vi "EDIT USER IN PGSQL.vi"(8 "USER/ITEM DATA TRANSFER IN":T2(array[cluster]), 9 "REFERENCES":T3, 10 "USER INFO IN":T4, 11 "Image In":T1) -> (0 "USER/ITEM DATA TRANSFER OUT":T2(array[cluster]), 2 "USER INFO OUT":T4)   [LabVIEW 2019]
uses:
  Controls/References Cluster.ctl
  <vilib>/userDefined/High Color/IMAQdx.ctl
  Controls/Custom Calendar/Custom Calendar.xctl
  <vilib>/vision/Image Controls.llb/IMAQ Image.ctl
  Controls/Table Data Types/User Data Type.ctl
  <vilib>/addons/database/Connection.llb/DB Tools Open Connec (String).vi
  <vilib>/addons/database/Connection.llb/Conn Execute.vi
  <vilib>/addons/database/Recordset.llb/Rec Destroy - Connection.vi
  <vilib>/addons/database/NI_Database_API.lvlib
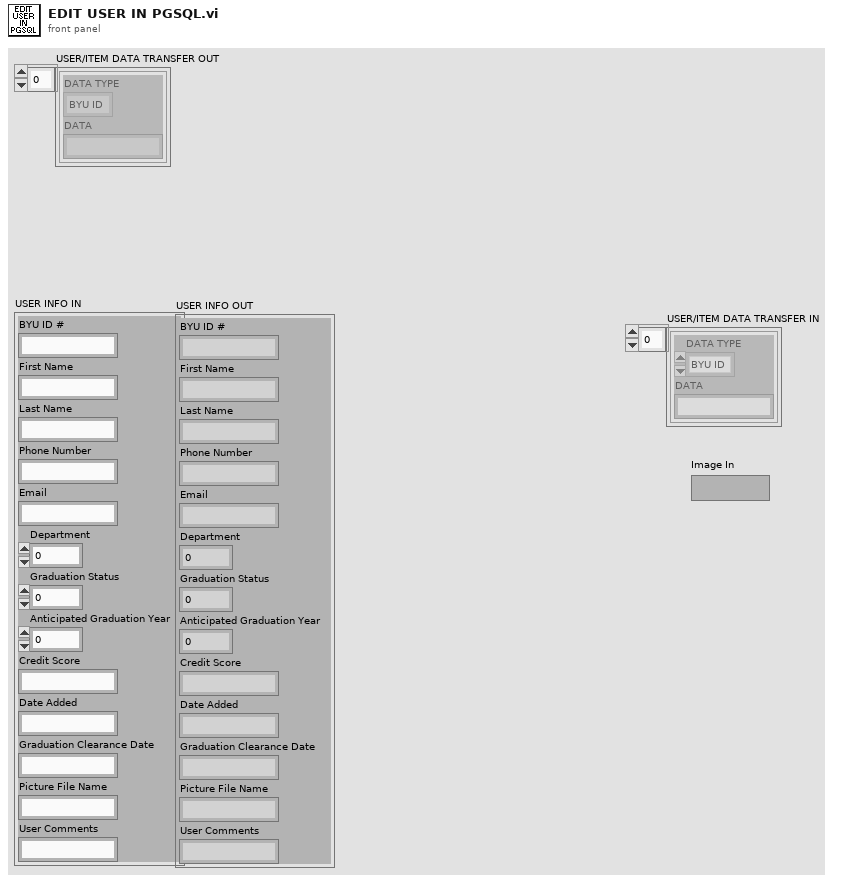
[diagram p1: front panel]
types:
  T1 = typedef "IMAQ Image.ctl" = refnum<image>
  T2 = cluster{"DATA TYPE":enum16{"BYU ID", "ME#/IDENTIFIER", "BYU ICN"}, "DATA":string}[]
  T3 = typedef "References Cluster.ctl" = cluster{"MAIN PAGES":refnum<vi>, "ADD/EDIT ITEM REFERENCES":cluster{"Identifier":refnum<vi>, "BYU ICN #":refnum<vi>, "Item Description":refnum<vi>, "Comments":refnum<vi>, "Checked Out Date":refnum<vi>, "Due Date":refnum<vi>, "Check Out Location":refnum<vi>, "Reminder Count":refnum<vi>, "Most Recent Reminder Date":refnum<vi>, "BYU ID #":refnum<vi>, "Building/Room":refnum<vi>, "Location in Room":refnum<vi>, "Manual":refnum<vi>, "Manufacturer":refnum<vi>, "Model #":refnum<vi>, "Serial #":refnum<vi>, "Date Acquired":refnum<vi>, "ADD/EDIT ITEM LABEL":refnum<vi>, "ARCHIVE ITEM":refnum<vi>, "Archive Item Inputs":refnum<vi>, "Reminder Notes":refnum<vi>}, "ADD/EDIT USER REFERENCES":cluster{"BYU ID # (##-###-####)":refnum<vi>, "First Name":refnum<vi>, "Last Name":refnum<vi>, "Phone Number (###-###-####)":refnum<vi>, "Email":refnum<vi>, "Department":refnum<vi>, "Graduation Status":refnum<vi>, "Anticipated Graduation Year":refnum<vi>, "Credit Score":refnum<vi>, "Date Added":refnum<vi>, "Graduation Clearance Date":refnum<vi>, "Picture File Name":refnum<vi>, "ADD/EDIT USER LABEL":refnum<vi>, "Department Map":refnum<vi>, "Status Map":refnum<vi>, "Anticipated Graduation Year Map":refnum<vi>, "User Agreement":refnum<vi>, "User Comments":refnum<vi>, "Camera":refnum<vi>}, "RETURN ITEM REFERENCES":cluster{"Item or Person:":refnum<vi>, "Search Return Results":refnum<vi>, "What are you searching for?":refnum<vi>}, "SEARCH DATABASE REFERENCES":cluster{"What to Search For:":refnum<vi>, "Where to Search":refnum<vi>, "Column to Search In":refnum<vi>, "Column to Sort By":refnum<vi>, "Search Database Results":refnum<vi>, "Inventory Column Selector":refnum<vi>, "User Column Selector":refnum<vi>, "Inventory Archive Column Selector":refnum<vi>, "User Archive Column Selector":refnum<vi>, "Sales Tracking Column Selector":refnum<vi>, "Checked In Archive Column Selector":refnum<vi>, "Restore User":refnum<vi>, "Date Range":refnum<vi>, "Dates Less Than":refnum<vi>, "Dates Greater Than":refnum<vi>, "Search Print Receipt":refnum<vi>}, "USER ITEMS REFERENCES":cluster{"USER'S INFORMATION":refnum<vi>, "User's Checked Out Items":refnum<vi>, "User Info Comments":refnum<vi>, "SEE USER INFO COMMENTS":refnum<vi>}, "EDIT ITEMS REFERENCES":cluster{"New Check Out Location":refnum<vi>, "Items to Edit":refnum<vi>, "Edit Items Due Date":refnum<vi>, "New Reminder Notes":refnum<vi>, "New Item Description":refnum<vi>}, "CHECK OUT ITEMS REFERENCES":cluster{"Enter Item:":refnum<vi>, "Check Out Items Due Date":refnum<vi>, "Check Out Location":refnum<vi>, "Items to be Checked Out":refnum<vi>, "Possible Items":refnum<vi>}, "TRANSFER ITEMS REFERENCES":cluster{"Search Parameter":refnum<vi>, "What to Match":refnum<vi>, "Matching Individuals":refnum<vi>, "Items to be Transferred":refnum<vi>}, "SETTINGS REFERENCES":cluster{"PSC Database Settings":refnum<vi>, "PSC Sales Item Spreadsheet":refnum<vi>}, "PSC SALES REFERENCES":cluster{"BYU ID CARD #":refnum<vi>, "Sale Description":refnum<vi>, "Scan or Enter Item Name":refnum<vi>, "Items to be Sold":refnum<vi>, "Grand Total":refnum<vi>, "Item List":refnum<vi>}}
  T4 = cluster{"BYU ID #":string, "First Name":string, "Last Name":string, "Phone Number":string, "Email":string, "Department":u16, "Graduation Status":u16, "Anticipated Graduation Year":u16, "Credit Score":string, "Date Added":string, "Graduation Clearance Date":string, "Picture File Name":string, "User Comments":string}
  T5 = typedef "User Data Type.ctl" = cluster{"BYU ID #":string, "First Name":string, "Last Name":string, "Phone Number":string, "Email":string, "Department":string, "Graduation Status":string, "Anticipated Graduation Year":string, "Credit Score":dbl, "Date Added":string, "Graduation Clearance Date":string, "Picture File Name":string, "User Comments":string}
  T6 = cluster{"BYU ID # (##-###-####)":refnum<vi>, "First Name":refnum<vi>, "Last Name":refnum<vi>, "Phone Number (###-###-####)":refnum<vi>, "Email":refnum<vi>, "Department":refnum<vi>, "Graduation Status":refnum<vi>, "Anticipated Graduation Year":refnum<vi>, "Credit Score":refnum<vi>, "Date Added":refnum<vi>, "Graduation Clearance Date":refnum<vi>, "Picture File Name":refnum<vi>, "ADD/EDIT USER LABEL":refnum<vi>, "Department Map":refnum<vi>, "Status Map":refnum<vi>, "Anticipated Graduation Year Map":refnum<vi>, "User Agreement":refnum<vi>, "User Comments":refnum<vi>, "Camera":refnum<vi>}
  T7 = cluster{"DATA TYPE":enum16{"BYU ID", "ME#/IDENTIFIER", "BYU ICN"}, "DATA":string}
  T8 = typedef "NI_Database_API.lvlib/Conn ObjectReference.ctl" = refnum<k1>
  T9 = typedef "NI_Database_API.lvlib/Rec ObjectReference.ctl" = refnum<k1>
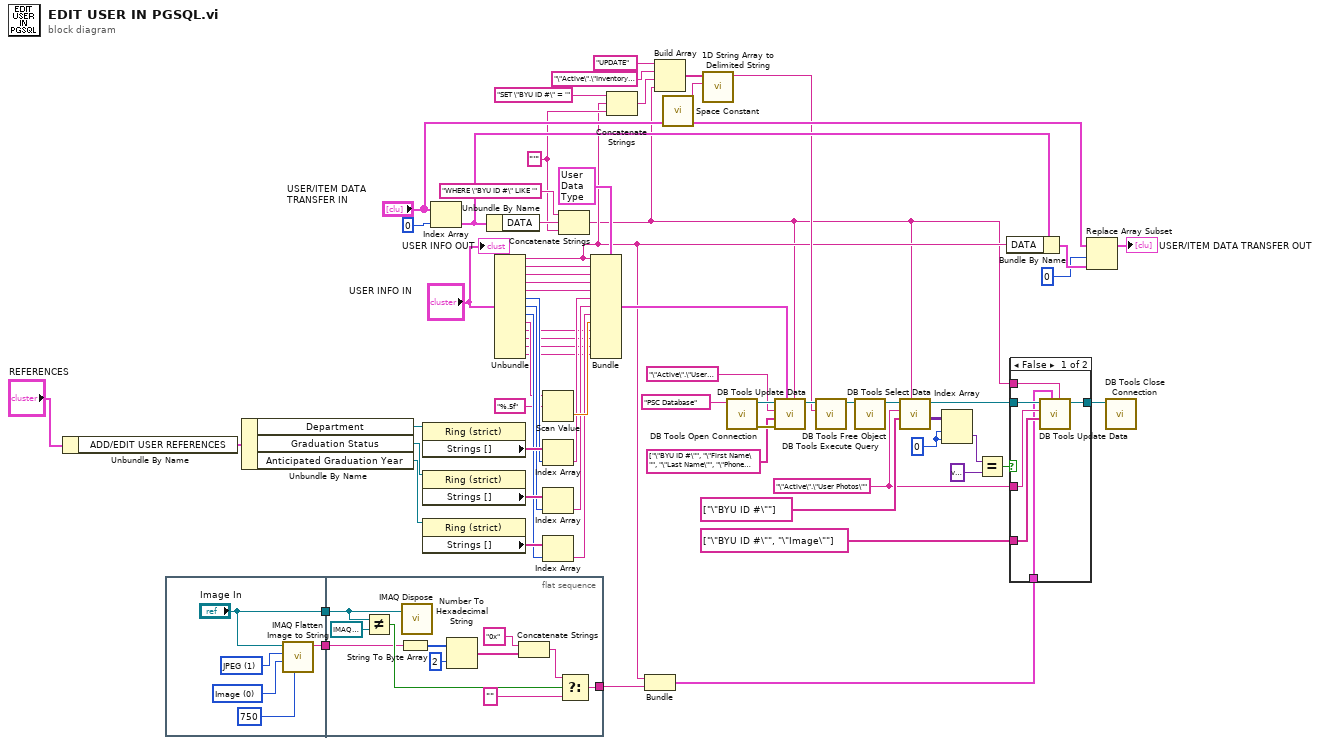
[diagram p0: block diagram]
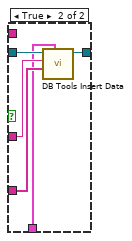
[diagram p2: hidden frame]
diagram:
  w13 = 0 ("disabled index (col)")
  w7 = "\"Active\".\"User Photos\"" ("table")
  w25 = "'" ("string")
  n1 = Unbundle By Name("REFERENCES") -> ("ADD/EDIT USER REFERENCES"=w62:T6)
  n2 = flat-sequence {
    tunnel: ["Image In"] -> w17
    tunnel: [w69] -> w16
    tunnel: w17 -> [w83]
    tunnel: w16 -> [w76]
    tunnel: [w74] -> w10
    frame #0 {
      w72 = 0 items=["Image", "Image and Vision Info", "Reference to Image"] ("Type of Flatten (Image and Vision Info)")
      w73 = 1 items=["None", "JPEG", "PACKED BINARY"] ("Compression (None)")
      n3 = call "IMAQ Flatten Image to String"("Quality (750)"=750, "Type of Flatten (Image and Vision Info)"=w72, "Compression (None)"=w73, "Image"="Image In") -> ("Data String"=w69:string)  [unwired: 6 in, 1 out]
    }
    frame #1 {
      n4 = Not Equal?(x=w83, y=T1 refnum) -> (x != y?=w82:bool)
      n5 = String To Byte Array(string=w76) -> (unsigned byte array=w80:u8[])
      n6 = call "IMAQ Dispose"("Image"=w83) -> ()  [unwired: 5 in, 1 out]
      n7 = Number To Hexadecimal String(1:i16 2 ("width (-)"), 2:w80) -> (0:w79:string[])
      n8 = Concatenate Strings("0x" ("string"), w79) -> (w75:string)
      n9 = Select(t=w75, s=w82, f="") -> (s? t:f=w74:string)
    }
  }
  n10 = Unbundle By Name(w62) -> ("Department"=w51:refnum<vi>, "Graduation Status"=w61:refnum<vi>, "Anticipated Graduation Year"=w60:refnum<vi>)
  n11 = property class="Ring (strict)"(reference=w51) -> ("Strings []"=w52:string[])  [unwired: 1 in, 2 out]
  n12 = property class="Ring (strict)"(reference=w61) -> ("Strings []"=w50:string[])  [unwired: 1 in, 2 out]
  n13 = property class="Ring (strict)"(reference=w60) -> ("Strings []"=w49:string[])  [unwired: 1 in, 2 out]
  n14 = Index Array(array="USER/ITEM DATA TRANSFER IN", index=0) -> (element=w33:T7)
  n15 = Unbundle By Name(w33) -> ("DATA"=w64:string)
  n16 = Unbundle("USER INFO IN") -> ("BYU ID #"=w9:string, "First Name"=w56:string, "Last Name"=w55:string, "Phone Number"=w54:string, "Email"=w53:string, "Department"=w48:u16, "Graduation Status"=w47:u16, "Anticipated Graduation Year"=w46:u16, "Credit Score"=w45:string, "Date Added"=w39:string, "Graduation Clearance Date"=w38:string, "Picture File Name"=w37:string, "User Comments"=w18:string)
  n17 = Scan Value(string=w45, format string="%.5f") -> (value=w43:dbl)  [unwired: 1 in, 1 out]
  n18 = Index Array(array=w52, index=w48) -> (element=w42:string)
  n19 = Index Array(array=w50, index=w47) -> (element=w41:string)
  n20 = Index Array(array=w49, index=w46) -> (element=w40:string)
  n21 = Concatenate Strings("WHERE \"BYU ID #\" LIKE '" ("string"), w64, w25) -> (w3:string)
  n22 = Bundle(cluster=T5 {"BYU ID #"="", "First Name"="", "Last Name"="", "Phone Number"="", "Email"="", "Department"="", "Graduation Status"="", "Anticipated Graduation Year"="", "Credit Score"=0.0, "Date Added"="", "Graduation Clearance Date"="", "Picture File Name"="", "User Comments"=""} ("USER DATA TYPE"), "BYU ID #"=w9, "First Name"=w56, "Last Name"=w55, "Phone Number"=w54, "Email"=w53, "Department"=w42, "Graduation Status"=w41, "Anticipated Graduation Year"=w40, "Credit Score"=w43, "Date Added"=w39, "Graduation Clearance Date"=w38, "Picture File Name"=w37, "User Comments"=w18) -> (w36:T5)
  n23 = Concatenate Strings("SET \"BYU ID #\" = '" ("string"), w9, w25) -> (w22:string)
  n24 = Bundle("BYU ID #"=w9, "f"=w10) -> (w5:cluster{"BYU ID #":string, "f":string})  [unwired: 1 in]
  n25 = Build Array("UPDATE" ("string"), "\"Active\".\"Inventory\"" ("table"), w22, w3) -> (w21:string[])
  n26 = call <vilib>:"Space Constant.vi"() -> ("String"=w20:string)
  n27 = call <vilib>:"1D String Array to Delimited String.vi"("delimiter"=w20, "string array"=w21) -> ("delimited string"=w19:string)  [unwired: 9 in]
  n28 = call-poly <vilib>:"DB Tools Open Connection.vi"("connection information"="PSC Database" ("table")) -> ("error out"=w67:errorcluster, "connection reference"=w68:T8)  [unwired: 7 in]
  n29 = call <vilib>:"DB Tools Update Data.vi"("condition"=w3, "data"=w36, "error in (no error)"=w67, "columns"=string[] ["\"BYU ID #\"", "\"First Name\"", "\"Last Name\"", "\"Phone Number\"", "\"Email\"", "\"Department\"", "\"Graduation Status\"", "\"Anticipated Graduation Year\"", "\"Credit Score\"", "\"Date Added\"", "\"Graduation Clearance Date\"", "\"Picture File Name\"", "\"Comments\""], "table"="\"Active\".\"Users\"", "connection reference"=w68) -> ("connection reference out"=w28:T8)  [unwired: 4 in, 1 out]
  n30 = call-poly <vilib>:"DB Tools Execute Query.vi"("SQL query"=w19, "connection reference"=w28) -> ("recordset reference"=w27:T9)  [unwired: 6 in, 1 out]
  n31 = call-poly <vilib>:"DB Tools Free Object.vi"("recordset reference"=w27) -> ("connection reference"=w15:T8)  [unwired: 9 in, 1 out]
  n32 = call <vilib>:"DB Tools Select Data.vi"("condition"=w3, "columns"=string[] ["\"BYU ID #\""], "table"=w7, "connection reference"=w15) -> ("data"=w12:variant[][], "connection reference out"=w8:T8)  [unwired: 2 in, 1 out]
  n33 = Index Array(array=w12, index (row)=w13, index (col)=w13) -> (element=w1:variant)
  n34 = Equal?(x=w1, y=variant) -> (x = y?=w11:bool)
  n35 = Bundle By Name(cluster=w33, "DATA"=w9) -> (w30:T7)
  n36 = case shown="False" w11 {
    tunnel: w8 -> [w90 w95]
    tunnel: w7 -> [w89 w94]
    tunnel: string[] ["\"BYU ID #\"", "\"Image\""] ("columns") -> [w88 w93]
    tunnel: w5 -> [w87 w92]
    tunnel: [w85 w91] -> w4
    tunnel: w3 -> [w86 _]
    frame False {
      n37 = call <vilib>:"DB Tools Update Data.vi"("condition"=w86, "data"=w87, "columns"=w88, "table"=w89, "connection reference"=w90) -> ("connection reference out"=w85:T8)  [unwired: 5 in, 1 out]
    }
    frame True {
      n38 = call <vilib>:"DB Tools Insert Data.vi"("data"=w92, "columns"=w93, "table"=w94, "connection reference"=w95) -> ("connection reference out"=w91:T8)  [unwired: 6 in, 1 out]
    }
  }
  n39 = Replace Array Subset(array="USER/ITEM DATA TRANSFER IN", new element=w30, index=0) -> (→"USER/ITEM DATA TRANSFER OUT":T2)
  n40 = call <vilib>:"DB Tools Close Connection.vi"("connection reference"=w4) -> ()  [unwired: 6 in, 1 out]
  "USER INFO OUT" <- "USER INFO IN"
